vi "bmp085_get_temperature.vi"(8 "error in (no error)":errorcluster, 11 "BMP085 (GY-65) in":refnum<class "BMP085 (GY-65).lvclass">) -> (0 "error out":errorcluster, 2 "T":i32, 3 "BMP085 (GY-65) out":refnum<class "BMP085 (GY-65).lvclass">)   [LabVIEW 2015, in "BMP085 (RT).lvlib" / "BMP085 (GY-65).lvclass"]
uses:
  BMP085 (GY-65).lvclass
  BMP085 (GY-65).lvclass/BMP085 (GY-65).ctl
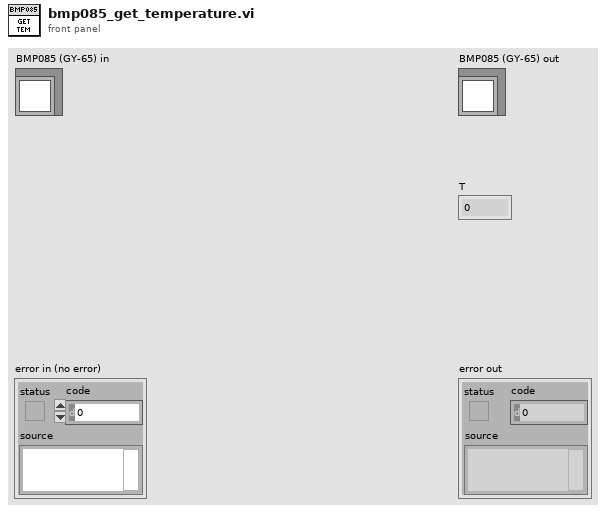
[diagram p1: front panel]
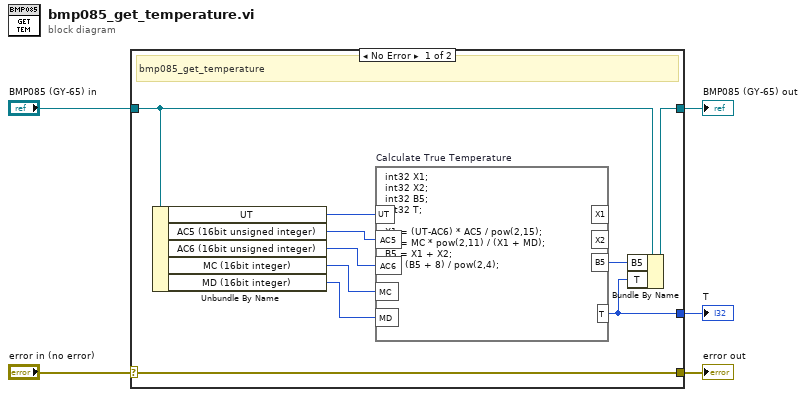
[diagram p0: block diagram]
diagram:
  n1 = case shown="No Error" "error in (no error)" {
    selector: "error in (no error)" -> [w15 w17]
    tunnel: [w15 w17] -> w4
    tunnel: [w8 w16] -> w2
    tunnel: "BMP085 (GY-65) in" -> [w14 w16]
    tunnel: [w7 _] -> w1
    frame No Error {
      # "bmp085_get_temperature"
      n2 = Unbundle By Name(w14) -> ("UT"=w13:i32, "AC5 (16bit unsigned integer)"=w12:u16, "AC6 (16bit unsigned integer)"=w11:u16, "MC (16bit integer)"=w10:i16, "MD (16bit integer)"=w9:i16)
      n3 = formula code="int32 X1;\nint32 X2;\nint32 B5;\nint32 T;\n\nX1 = (UT-AC6) * AC5 / pow(2,15);\nX2 = MC * pow(2,11) / (X1 + MD);\nB5 = X1 + X2;\nT = (B5 + 8) / pow(2,4);" "Calculate True Temperature"("UT"=w13, "AC6"=w11, "AC5"=w12, "MC"=w10, "MD"=w9) -> ("B5"=w6:i32, "T"=w7:i32)  [unwired: 2 out]
      n4 = Bundle By Name(cluster=w14, "B5"=w6, "T"=w7) -> (w8:refnum<class "BMP085 (GY-65).lvclass">)
    }
    frame Error {
    }
  }
  "error out" <- w4
  "BMP085 (GY-65) out" <- w2
  "T" <- w1
